vi "Autotest.vi"(8 "error in (no error)":errorcluster caption="entrée d'erreur (pas d'erreur)", 11 "Class Relay_Board usb_relay_device en entrée":refnum<class "Class Relay_Board usb_Relay_device.lvclass">) -> (0 "error out":errorcluster caption="sortie d'erreur", 2 "Autotest Ok ?":bool, 3 "Class Relay_Board usb_relay_device en sortie":refnum<class "Class Relay_Board usb_Relay_device.lvclass">)   [LabVIEW 2020, in "Library Instrument & Equipement.lvlib" / "Library Relay_Board.lvlib" / "Class Relay_Board usb_Relay_device.lvclass"]
uses:
  Class Relay_Board usb_Relay_device.lvclass
  Class Relay_Board usb_Relay_device.lvclass/Class Relay_Board usb_Relay_device.ctl
  usb_relay_device/usb_relay_device.lvlib
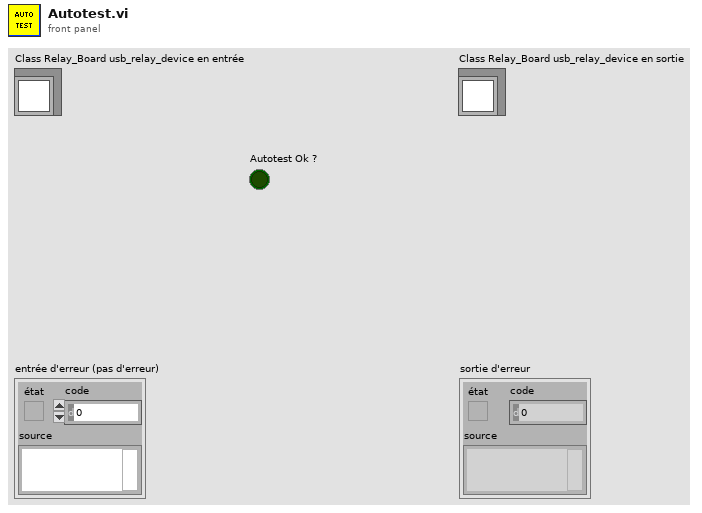
[diagram p1: front panel]
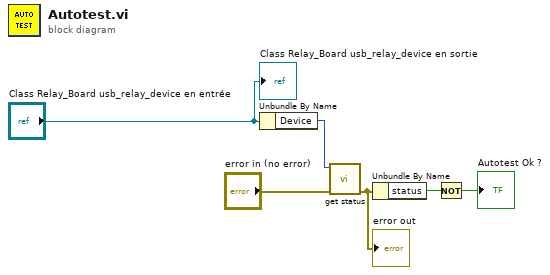
[diagram p0: block diagram]
diagram:
  n1 = Unbundle By Name("Class Relay_Board usb_relay_device en entrée") -> ("Device"=w6:i32)
  n2 = call "get status.vi"("error in (no error)"="error in (no error)", "hHandle"=w6) -> ("error out"=w4:errorcluster)  [unwired: 8 in, 1 out]
  "error out" <- w4
  n3 = Unbundle By Name(w4) -> ("status"=w3:bool)
  n4 = Not(x=w3) -> (.not. x?=→"Autotest Ok ?":bool)
  "Class Relay_Board usb_relay_device en sortie" <- "Class Relay_Board usb_relay_device en entrée"
